vi "VISJS Viewer.vi"(4 "Extra Scripts":string, 5 "FileDependency out":map{path, T1}(c390), 6 "Options":string, 7 "OpenWebBrowser(False)":bool, 8 "error in":errorcluster, 9 "Embedd VISJS Librarya in HTMl File(False)":bool, 10 "HTMLFilePath":path, 11 "LibraryDependency":map{path, T3}(c390)) -> (0 "error out":errorcluster, 3 "HTMLFileContent":string)   [LabVIEW 2020, in "VISJS Viewer.lvlib"] (continued)
;case 7:g.next=3;break;case 9:g.next=14;break;case 11:g.prev=11,g.t0=g.catch(1),t.e(g.t0);case 14:return g.prev=14,t.f(),g.finish(14);case 17:case\"end\":return g.stop()}}),g,this,[[1,11,14,17]])}))},{key:\"keys\",value:TE.mark((function g(){var t,A,e,C;return TE.wrap((function(g){for(;;)switch(g.prev=g.next){case 0:t=hD(this._pairs),g.prev=1,t.s();case 3:if((A=t.n()).done){g.next=9;break}return e=lh(A.value,1),C=e[0],g.next=7,C;case 7:g.next=3;break;case 9:g.next=14;break;case 11:g.prev=11,g.t0=g.catch(1),t.e(g.t0);case 14:return g.prev=14,t.f(),g.finish(14);case 17:case\"end\":return g.stop()}}),g,this,[[1,11,14,17]])}))},{key:\"values\",value:TE.mark((function g(){var t,A,e,C;return TE.wrap((function(g){for(;;)switch(g.prev=g.next){case 0:t=hD(this._pairs),g.prev=1,t.s();case 3:if((A=t.n()).done){g.next=9;break}return e=lh(A.value,2),C=e[1],g.next=7,C;case 7:g.next=3;break;case 9:g.next=14;break;case 11:g.prev=11,g.t0=g.catch(1),t.e(g.t0);case 14:return g.prev=14,t.f(),g.finish(14);case 17:case\"end\":return g.stop()}}),g,this,[[1,11,14,17]])}))},{key:\"toIdArray\",value:function(){var g;return Fh(g=ch(this._pairs)).call(g,(function(g){return g[0]}))}},{key:\"toItemArray\",value:function(){var g;return Fh(g=ch(this._pairs)).call(g,(function(g){return g[1]}))}},{key:\"toEntryArray\",value:function(){return ch(this._pairs)}},{key:\"toObjectMap\",value:function(){var g,t=$c(null),A=hD(this._pairs);try{for(A.s();!(g=A.n()).done;){var e=lh(g.value,2),C=e[0],I=e[1];t[C]=I}}catch(g){A.e(g)}finally{A.f()}return t}},{key:\"toMap\",value:function(){return new Fm(this._pairs)}},{key:\"toIdSet\",value:function(){return new CO(this.toIdArray())}},{key:\"toItemSet\",value:function(){return new CO(this.toItemArray())}},{key:\"cache\",value:function(){return new g(ch(this._pairs))}},{key:\"distinct\",value:function(g){var t,A=new CO,e=hD(this._pairs);try{for(e.s();!(t=e.n()).done;){var C=lh(t.value,2),I=C[0],i=C[1];A.add(g(i,I))}}catch(g){e.e(g)}finally{e.f()}return A}},{key:\"filter\",value:function(t){var A=this._pairs;return new g(rb({},IO,TE.mark((function g(){var e,C,I,i,o;return TE.wrap((function(g){for(;;)switch(g.prev=g.next){case 0:e=hD(A),g.prev=1,e.s();case 3:if((C=e.n()).done){g.next=10;break}if(I=lh(C.value,2),i=I[0],o=I[1],!t(o,i)){g.next=8;break}return g.next=8,[i,o];case 8:g.next=3;break;case 10:g.next=15;break;case 12:g.prev=12,g.t0=g.catch(1),e.e(g.t0);case 15:return g.prev=15,e.f(),g.finish(15);case 18:case\"end\":return g.stop()}}),g,null,[[1,12,15,18]])}))))}},{key:\"forEach\",value:function(g){var t,A=hD(this._pairs);try{for(A.s();!(t=A.n()).done;){var e=lh(t.value,2),C=e[0];g(e[1],C)}}catch(g){A.e(g)}finally{A.f()}}},{key:\"map\",value:function(t){var A=this._pairs;return new g(rb({},IO,TE.mark((function g(){var e,C,I,i,o;return TE.wrap((function(g){for(;;)switch(g.prev=g.next){case 0:e=hD(A),g.prev=1,e.s();case 3:if((C=e.n()).done){g.next=9;break}return I=lh(C.value,2),i=I[0],o=I[1],g.next=7,[i,t(o,i)];case 7:g.next=3;break;case 9:g.next=14;break;case 11:g.prev=11,g.t0=g.catch(1),e.e(g.t0);case 14:return g.prev=14,e.f(),g.finish(14);case 17:case\"end\":return g.stop()}}),g,null,[[1,11,14,17]])}))))}},{key:\"max\",value:function(g){var t=iO(this._pairs),A=t.next();if(A.done)return null;for(var e=A.value[1],C=g(A.value[1],A.value[0]);!(A=t.next()).done;){var I=lh(A.value,2),i=I[0],o=I[1],n=g(o,i);n>C&&(C=n,e=o)}return e}},{key:\"min\",value:function(g){var t=iO(this._pairs),A=t.next();if(A.done)return null;for(var e=A.value[1],C=g(A.value[1],A.value[0]);!(A=t.next()).done;){var I=lh(A.value,2),i=I[0],o=I[1],n=g(o,i);n<C&&(C=n,e=o)}return e}},{key:\"reduce\",value:function(g,t){var A,e=hD(this._pairs);try{for(e.s();!(A=e.n()).done;){var C=lh(A.value,2),I=C[0];t=g(t,C[1],I)}}catch(g){e.e(g)}finally{e.f()}return t}},{key:\"sort\",value:function(t){var A=this;return new g(rb({},IO,(function(){var g;return iO(WO(g=ch(A._pairs)).call(g,(function(g,A){var e=lh(g,2),C=e[0],I=e[1],i=lh(A,2),o=i[0],n=i[1];return t(I,n,C,o)})))})))}}]),g}();var mD=function(g){Cb(A,g);var t=dD(A);function A(g,e){var C;return cn(this,A),rb(Jm(C=t.call(this)),\"flush\",void 0),rb(Jm(C),\"length\",void 0),rb(Jm(C),\"_options\",void 0),rb(Jm(C),\"_data\",void 0),rb(Jm(C),\"_idProp\",void 0),rb(Jm(C),\"_queue\",null),g&&!Rh(g)&&(e=g,g=[]),C._options=e||{},C._data=new Fm,C.length=0,C._idProp=C._options.fieldId||\"id\",g&&g.length&&C.add(g),C.setOptions(e),C}return kd(A,[{key:\"idProp\",get:function(){return this._idProp}},{key:\"setOptions\",value:function(g){g&&void 0!==g.queue&&(!1===g.queue?this._queue&&(this._queue.destroy(),this._queue=null):(this._queue||(this._queue=fD.extend(this,{replace:[\"add\",\"update\",\"remove\"]})),g.queue&&\"object\"===yd(g.queue)&&this._queue.setOptions(g.queue)))}},{key:\"add\",value:function(g,t){var A,e=this,C=[];if(Rh(g)){var I=Fh(g).call(g,(function(g){return g[e._idProp]}));if(Xm(I).call(I,(function(g){return e._data.has(g)})))throw new Error(\"A duplicate id was found in the parameter array.\");for(var i=0,o=g.length;i<o;i++)A=this._addItem(g[i]),C.push(A)}else{if(!g||\"object\"!==yd(g))throw new Error(\"Unknown dataType\");A=this._addItem(g),C.push(A)}return C.length&&this._trigger(\"add\",{items:C},t),C}},{key:\"update\",value:function(g,t){var A=this,e=[],C=[],I=[],i=[],o=this._idProp,n=function(g){var t=g[o];if(null!=t&&A._data.has(t)){var n=g,r=fe({},A._data.get(t)),s=A._updateItem(n);C.push(s),i.push(n),I.push(r)}else{var a=A._addItem(g);e.push(a)}};if(Rh(g))for(var r=0,s=g.length;r<s;r++)g[r]&&\"object\"===yd(g[r])?n(g[r]):console.warn(\"Ignoring input item, which is not an object at index \"+r);else{if(!g||\"object\"!==yd(g))throw new Error(\"Unknown dataType\");n(g)}if(e.length&&this._trigger(\"add\",{items:e},t),C.length){var a={items:C,oldData:I,data:i};this._trigger(\"update\",a,t)}return bh(e).call(e,C)}},{key:\"updateOnly\",value:function(g,t){var A,e=this;Rh(g)||(g=[g]);var C=Fh(A=Fh(g).call(g,(function(g){var t=e._data.get(g[e._idProp]);if(null==t)throw new Error(\"Updating non-existent items is not allowed.\");return{oldData:t,update:g}}))).call(A,(function(g){var t=g.oldData,A=g.update,C=t[e._idProp],I=function(g){for(var t,A=arguments.length,e=new Array(A>1?A-1:0),C=1;C<A;C++)e[C-1]=arguments[C];return Bf.apply(void 0,bh(t=[{},g]).call(t,e))}(t,A);return e._data.set(C,I),{id:C,oldData:t,updatedData:I}}));if(C.length){var I={items:Fh(C).call(C,(function(g){return g.id})),oldData:Fh(C).call(C,(function(g){return g.oldData})),data:Fh(C).call(C,(function(g){return g.updatedData}))};return this._trigger(\"update\",I,t),I.items}return[]}},{key:\"get\",value:function(g,t){var A=void 0,e=void 0,C=void 0;pD(g)?(A=g,C=t):Rh(g)?(e=g,C=t):C=g;var I,i=C&&\"Object\"===C.returnType?\"Object\":\"Array\",o=C&&pc(C),n=[],r=void 0,s=void 0,a=void 0;if(null!=A)(r=this._data.get(A))&&o&&!o(r)&&(r=void 0);else if(null!=e)for(var d=0,h=e.length;d<h;d++)null==(r=this._data.get(e[d]))||o&&!o(r)||n.push(r);else for(var l,c=0,u=(s=ch($O(l=this._data).call(l))).length;c<u;c++)a=s[c],null==(r=this._data.get(a))||o&&!o(r)||n.push(r);if(C&&C.order&&null==A&&this._sort(n,C.order),C&&C.fields){var p=C.fields;if(null!=A&&null!=r)r=this._filterFields(r,p);else for(var f=0,v=n.length;f<v;f++)n[f]=this._filterFields(n[f],p)}if(\"Object\"==i){for(var y={},m=0,b=n.length;m<b;m++){var w=n[m];y[w[this._idProp]]=w}return y}return null!=A?null!==(I=r)&&void 0!==I?I:null:n}},{key:\"getIds\",value:function(g){var t=this._data,A=g&&pc(g),e=g&&g.order,C=ch($O(t).call(t)),I=[];if(A)if(e){for(var i=[],o=0,n=C.length;o<n;o++){var r=C[o],s=this._data.get(r);null!=s&&A(s)&&i.push(s)}this._sort(i,e);for(var a=0,d=i.length;a<d;a++)I.push(i[a][this._idProp])}else for(var h=0,l=C.length;h<l;h++){var c=C[h],u=this._data.get(c);null!=u&&A(u)&&I.push(u[this._idProp])}else if(e){for(var p=[],f=0,v=C.length;f<v;f++){var y=C[f];p.push(t.get(y))}this._sort(p,e);for(var m=0,b=p.length;m<b;m++)I.push(p[m][this._idProp])}else for(var w=0,k=C.length;w<k;w++){var x=C[w],E=t.get(x);null!=E&&I.push(E[this._idProp])}return I}},{key:\"getDataSet\",value:function(){return this}},{key:\"forEach\",value:function(g,t){var A=t&&pc(t),e=this._data,C=ch($O(e).call(e));if(t&&t.order)for(var I=this.get(t),i=0,o=I.length;i<o;i++){var n=I[i];g(n,n[this._idProp])}else for(var r=0,s=C.length;r<s;r++){var a=C[r],d=this._data.get(a);null==d||A&&!A(d)||g(d,a)}}},{key:\"map\",value:function(g,t){for(var A=t&&pc(t),e=[],C=this._data,I=ch($O(C).call(C)),i=0,o=I.length;i<o;i++){var n=I[i],r=this._data.get(n);null==r||A&&!A(r)||e.push(g(r,n))}return t&&t.order&&this._sort(e,t.order),e}},{key:\"_filterFields\",value:function(g,t){var A;return g?LE(A=Rh(t)?t:Lh(t)).call(A,(function(t,A){return t[A]=g[A],t}),{}):g}},{key:\"_sort\",value:function(g,t){if(\"string\"==typeof t){var A=t;WO(g).call(g,(function(g,t){var e=g[A],C=t[A];return e>C?1:e<C?-1:0}))}else{if(\"function\"!=typeof t)throw new TypeError(\"Order must be a function or a string\");WO(g).call(g,t)}}},{key:\"remove\",value:function(g,t){for(var A=[],e=[],C=Rh(g)?g:[g],I=0,i=C.length;I<i;I++){var o=this._remove(C[I]);if(o){var n=o[this._idProp];null!=n&&(A.push(n),e.push(o))}}return A.length&&this._trigger(\"remove\",{items:A,oldData:e},t),A}},{key:\"_remove\",value:function(g){var t;if(pD(g)?t=g:g&&\"object\"===yd(g)&&(t=g[this._idProp]),null!=t&&this._data.has(t)){var A=this._data.get(t)||null;return this._data.delete(t),--this.length,A}return null}},{key:\"clear\",value:function(g){for(var t,A=ch($O(t=this._data).call(t)),e=[],C=0,I=A.length;C<I;C++)e.push(this._data.get(A[C]));return this._data.clear(),this.length=0,this._trigger(\"remove\",{items:A,oldData:e},g),A}},{key:\"max\",value:function(g){var t,A,e=null,C=null,I=hD(nT(t=this._data).call(t));try{for(I.s();!(A=I.n()).done;){var i=A.value,o=i[g];\"number\"==typeof o&&(null==C||o>C)&&(e=i,C=o)}}catch(g){I.e(g)}finally{I.f()}return e||null}},{key:\"min\",value:function(g){var t,A,e=null,C=null,I=hD(nT(t=this._data).call(t));try{for(I.s();!(A=I.n()).done;){var i=A.value,o=i[g];\"number\"==typeof o&&(null==C||o<C)&&(e=i,C=o)}}catch(g){I.e(g)}finally{I.f()}return e||null}},{key:\"distinct\",value:function(g){for(var t=this._data,A=ch($O(t).call(t)),e=[],C=0,I=0,i=A.length;I<i;I++){for(var o=A[I],n=t.get(o)[g],r=!1,s=0;s<C;s++)if(e[s]==n){r=!0;break}r||void 0===n||(e[C]=n,C++)}return e}},{key:\"_addItem\",value:function(g){var t=function(g,t){return null==g[t]&&(g[t]=rD()),g}(g,this._idProp),A=t[this._idProp];if(this._data.has(A))throw new Error(\"Cannot add item: item with id \"+A+\" already exists\");return this._data.set(A,t),++this.length,A}},{key:\"_updateItem\",value:function(g){var t=g[this._idProp];if(null==t)throw new Error(\"Cannot update item: item has no id (item: \"+eu(g)+\")\");var A=this._data.get(t);if(!A)throw new Error(\"Cannot update item: no item with id \"+t+\" found\");return this._data.set(t,aD(aD({},A),g)),t}},{key:\"stream\",value:function(g){if(g){var t=this._data;return new yD(rb({},IO,TE.mark((function A(){var e,C,I,i;return TE.wrap((function(A){for(;;)switch(A.prev=A.next){case 0:e=hD(g),A.prev=1,e.s();case 3:if((C=e.n()).done){A.next=11;break}if(I=C.value,null==(i=t.get(I))){A.next=9;break}return A.next=9,[I,i];case 9:A.next=3;break;case 11:A.next=16;break;case 13:A.prev=13,A.t0=A.catch(1),e.e(A.t0);case 16:return A.prev=16,e.f(),A.finish(16);case 19:case\"end\":return A.stop()}}),A,null,[[1,13,16,19]])}))))}var A;return new yD(rb({},IO,je(A=pT(this._data)).call(A,this._data)))}}]),A}(vD),bD=function(g){Cb(A,g);var t=dD(A);function A(g,e){var C,I;return cn(this,A),rb(Jm(I=t.call(this)),\"length\",0),rb(Jm(I),\"_listener\",void 0),rb(Jm(I),\"_data\",void 0),rb(Jm(I),\"_ids\",new CO),rb(Jm(I),\"_options\",void 0),I._options=e||{},I._listener=je(C=I._onEvent).call(C,Jm(I)),I.setData(g),I}return kd(A,[{key:\"idProp\",get:function(){return this.getDataSet().idProp}},{key:\"setData\",value:function(g){if(this._data){this._data.off&&this._data.off(\"*\",this._listener);var t=this._data.getIds({filter:pc(this._options)}),A=this._data.get(t);this._ids.clear(),this.length=0,this._trigger(\"remove\",{items:t,oldData:A})}if(null!=g){this._data=g;for(var e=this._data.getIds({filter:pc(this._options)}),C=0,I=e.length;C<I;C++){var i=e[C];this._ids.add(i)}this.length=e.length,this._trigger(\"add\",{items:e})}else this._data=new mD;this._data.on&&this._data.on(\"*\",this._listener)}},{key:\"refresh\",value:function(){for(var g=this._data.getIds({filter:pc(this._options)}),t=ch(this._ids),A={},e=[],C=[],I=[],i=0,o=g.length;i<o;i++){var n=g[i];A[n]=!0,this._ids.has(n)||(e.push(n),this._ids.add(n))}for(var r=0,s=t.length;r<s;r++){var a=t[r],d=this._data.get(a);null==d?console.error(\"If you see this, report it please.\"):A[a]||(C.push(a),I.push(d),this._ids.delete(a))}this.length+=e.length-C.length,e.length&&this._trigger(\"add\",{items:e}),C.length&&this._trigger(\"remove\",{items:C,oldData:I})}},{key:\"get\",value:function(g,t){if(null==this._data)return null;var A,e=null;pD(g)||Rh(g)?(e=g,A=t):A=g;var C=fe({},this._options,A),I=pc(this._options),i=A&&pc(A);return I&&i&&(C.filter=function(g){return I(g)&&i(g)}),null==e?this._data.get(C):this._data.get(e,C)}},{key:\"getIds\",value:function(g){if(this._data.length){var t,A=pc(this._options),e=null!=g?pc(g):null;return t=e?A?function(g){return A(g)&&e(g)}:e:A,this._data.getIds({filter:t,order:g&&g.order})}return[]}},{key:\"forEach\",value:function(g,t){if(this._data){var A,e,C=pc(this._options),I=t&&pc(t);e=I?C?function(g){return C(g)&&I(g)}:I:C,Cl(A=this._data).call(A,g,{filter:e,order:t&&t.order})}}},{key:\"map\",value:function(g,t){if(this._data){var A,e,C=pc(this._options),I=t&&pc(t);return e=I?C?function(g){return C(g)&&I(g)}:I:C,Fh(A=this._data).call(A,g,{filter:e,order:t&&t.order})}return[]}},{key:\"getDataSet\",value:function(){return this._data.getDataSet()}},{key:\"stream\",value:function(g){var t;return this._data.stream(g||rb({},IO,je(t=$O(this._ids)).call(t,this._ids)))}},{key:\"dispose\",value:function(){var g;null!==(g=this._data)&&void 0!==g&&g.off&&this._data.off(\"*\",this._listener);var t,e=\"This data view has already been disposed of.\",C={get:function(){throw new Error(e)},set:function(){throw new Error(e)},configurable:!1},I=hD(Nh(A.prototype));try{for(I.s();!(t=I.n()).done;){var i=t.value;fT(this,i,C)}}catch(g){I.e(g)}finally{I.f()}}},{key:\"_onEvent\",value:function(g,t,A){if(t&&t.items&&this._data){var e=t.items,C=[],I=[],i=[],o=[],n=[],r=[];switch(g){case\"add\":for(var s=0,a=e.length;s<a;s++){var d=e[s];this.get(d)&&(this._ids.add(d),C.push(d))}break;case\"update\":for(var h=0,l=e.length;h<l;h++){var c=e[h];this.get(c)?this._ids.has(c)?(I.push(c),n.push(t.data[h]),o.push(t.oldData[h])):(this._ids.add(c),C.push(c)):this._ids.has(c)&&(this._ids.delete(c),i.push(c),r.push(t.oldData[h]))}break;case\"remove\":for(var u=0,p=e.length;u<p;u++){var f=e[u];this._ids.has(f)&&(this._ids.delete(f),i.push(f),r.push(t.oldData[u]))}}this.length+=C.length-i.length,C.length&&this._trigger(\"add\",{items:C},A),I.length&&this._trigger(\"update\",{items:I,oldData:o,data:n},A),i.length&&this._trigger(\"remove\",{items:i,oldData:r},A)}}}]),A}(vD);function wD(g,t){return\"object\"===yd(t)&&null!==t&&g===t.idProp&&\"function\"==typeof t.add&&\"function\"==typeof t.clear&&\"function\"==typeof t.distinct&&\"function\"==typeof Cl(t)&&\"function\"==typeof t.get&&\"function\"==typeof t.getDataSet&&\"function\"==typeof t.getIds&&\"number\"==typeof t.length&&\"function\"==typeof Fh(t)&&\"function\"==typeof t.max&&\"function\"==typeof t.min&&\"function\"==typeof t.off&&\"function\"==typeof t.on&&\"function\"==typeof t.remove&&\"function\"==typeof t.setOptions&&\"function\"==typeof t.stream&&\"function\"==typeof t.update&&\"function\"==typeof t.updateOnly}function kD(g,t){return\"object\"===yd(t)&&null!==t&&g===t.idProp&&\"function\"==typeof Cl(t)&&\"function\"==typeof t.get&&\"function\"==typeof t.getDataSet&&\"function\"==typeof t.getIds&&\"number\"==typeof t.length&&\"function\"==typeof Fh(t)&&\"function\"==typeof t.off&&\"function\"==typeof t.on&&\"function\"==typeof t.stream&&wD(g,t.getDataSet())}var xD=Object.freeze({__proto__:null,DELETE:Mf,DataSet:mD,DataStream:yD,DataView:bD,Queue:fD,createNewDataPipeFrom:function(g){return new uD(g)},isDataSetLike:wD,isDataViewLike:kD}),ED=C,OD=I,TD=sC,DD=Ec.trim,ND=fc,RD=u(\"\".charAt),PD=ED.parseFloat,MD=ED.Symbol,BD=MD&&MD.iterator,zD=1/PD(ND+\"-0\")!=-1/0||BD&&!OD((function(){PD(Object(BD))}))?function(g){var t=DD(TD(g)),A=PD(t);return 0===A&&\"-\"===RD(t,0)?-0:A}:PD;TA({global:!0,forced:parseFloat!==zD},{parseFloat:zD});var SD=A(tg.parseFloat),ZD=TA,FD=I,GD=er.f;ZD({target:\"Object\",stat:!0,forced:FD((function(){return!Object.getOwnPropertyNames(1)}))},{getOwnPropertyNames:GD});var jD=tg.Object,LD=function(g){return jD.getOwnPropertyNames(g)},VD=A(LD);function YD(g,t){var A=[\"node\",\"edge\",\"label\"],e=!0,C=lv(t,\"chosen\");if(\"boolean\"==typeof C)e=C;else if(\"object\"===yd(C)){if(-1===Xc(A).call(A,g))throw new Error(\"choosify: subOption '\"+g+\"' should be one of '\"+A.join(\"', '\")+\"'\");var I=lv(t,[\"chosen\",g]);\"boolean\"!=typeof I&&\"function\"!=typeof I||(e=I)}return e}function WD(g,t,A){if(g.width<=0||g.height<=0)return!1;if(void 0!==A){var e={x:t.x-A.x,y:t.y-A.y};if(0!==A.angle){var C=-A.angle;t={x:Math.cos(C)*e.x-Math.sin(C)*e.y,y:Math.sin(C)*e.x+Math.cos(C)*e.y}}else t=e}var I=g.x+g.width,i=g.y+g.width;return g.left<t.x&&I>t.x&&g.top<t.y&&i>t.y}function QD(g){return\"string\"==typeof g&&\"\"!==g}function UD(g,t,A,e){var C=e.x,I=e.y;if(\"function\"==typeof e.distanceToBorder){var i=e.distanceToBorder(g,t),o=Math.sin(t)*i,n=Math.cos(t)*i;n===i?(C+=i,I=e.y):o===i?(C=e.x,I-=i):(C+=n,I-=o)}else e.shape.width>e.shape.height?(C=e.x+.5*e.shape.width,I=e.y-A):(C=e.x+A,I=e.y-.5*e.shape.height);return{x:C,y:I}}var _D=function(){function g(t){cn(this,g),this.measureText=t,this.current=0,this.width=0,this.height=0,this.lines=[]}return kd(g,[{key:\"_add\",value:function(g,t){var A=arguments.length>2&&void 0!==arguments[2]?arguments[2]:\"normal\";void 0===this.lines[g]&&(this.lines[g]={width:0,height:0,blocks:[]});var e=t;void 0!==t&&\"\"!==t||(e=\" \");var C=this.measureText(e,A),I=fe({},nT(C));I.text=t,I.width=C.width,I.mod=A,void 0!==t&&\"\"!==t||(I.width=0),this.lines[g].blocks.push(I),this.lines[g].width+=I.width}},{key:\"curWidth\",value:function(){var g=this.lines[this.current];return void 0===g?0:g.width}},{key:\"append\",value:function(g){var t=arguments.length>1&&void 0!==arguments[1]?arguments[1]:\"normal\";this._add(this.current,g,t)}},{key:\"newLine\",value:function(g){var t=arguments.length>1&&void 0!==arguments[1]?arguments[1]:\"normal\";this._add(this.current,g,t),this.current++}},{key:\"determineLineHeights\",value:function(){for(var g=0;g<this.lines.length;g++){var t=this.lines[g],A=0;if(void 0!==t.blocks)for(var e=0;e<t.blocks.length;e++){var C=t.blocks[e];A<C.height&&(A=C.height)}t.height=A}}},{key:\"determineLabelSize\",value:function(){for(var g=0,t=0,A=0;A<this.lines.length;A++){var e=this.lines[A];e.width>g&&(g=e.width),t+=e.height}this.width=g,this.height=t}},{key:\"removeEmptyBlocks\",value:function(){for(var g=[],t=0;t<this.lines.length;t++){var A=this.lines[t];if(0!==A.blocks.length&&(t!==this.lines.length-1||0!==A.width)){var e={};fe(e,A),e.blocks=[];for(var C=void 0,I=[],i=0;i<A.blocks.length;i++){var o=A.blocks[i];0!==o.width?I.push(o):void 0===C&&(C=o)}0===I.length&&void 0!==C&&I.push(C),e.blocks=I,g.push(e)}}return g}},{key:\"finalize\",value:function(){this.determineLineHeights(),this.determineLabelSize();var g=this.removeEmptyBlocks();return{width:this.width,height:this.height,lines:g}}}]),g}(),KD={\"<b>\":/<b>/,\"<i>\":/<i>/,\"<code>\":/<code>/,\"</b>\":/<\\/b>/,\"</i>\":/<\\/i>/,\"</code>\":/<\\/code>/,\"*\":/\\*/,_:/_/,\"`\":/`/,afterBold:/[^*]/,afterItal:/[^_]/,afterMono:/[^`]/},HD=function(){function g(t){cn(this,g),this.text=t,this.bold=!1,this.ital=!1,this.mono=!1,this.spacing=!1,this.position=0,this.buffer=\"\"
